vi "RSNRPZ Revision Query.vi"(8 "error in (no error)":errorcluster, 11 "VISA session":refnum<visa-resource-name> caption="VISA resource name") -> (0 "error out":errorcluster, 1 "Firmware Revision":string, 2 "Instrument Driver Revision":string, 3 "dup VISA session":refnum<visa-resource-name> caption="VISA resource name")   [LabVIEW 2010]
doc: "This VI returns the DRIVER revision (only). Although a parameter for the INSTRUMENT revision exists, the instrument revision is NOT set by this function, but an empty string is always returned for the instrument revision"
uses:
  rsnrpz_32.dll
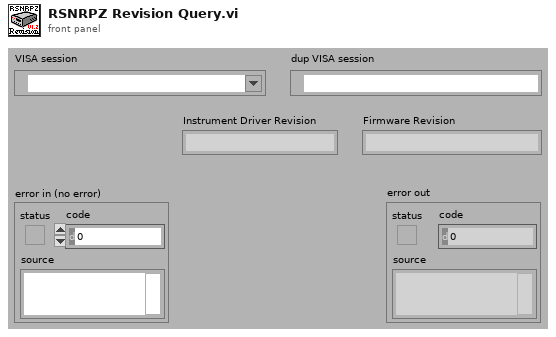
[diagram p1: front panel]
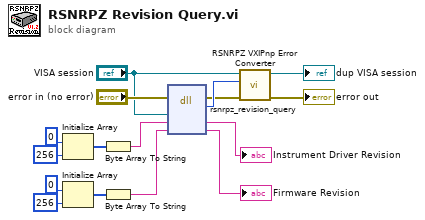
[diagram p0: block diagram]
diagram:
  n1 = Initialize Array(u8 0, 256) -> (w14:u8[])
  n2 = Initialize Array(u8 0, 256) -> (w11:u8[])
  n3 = Byte Array To String(unsigned byte array=w14) -> (string=w9:string)
  n4 = Byte Array To String(unsigned byte array=w11) -> (string=w7:string)
  n5 = dll-call lib="rsnrpz_32.dll" fn="rsnrpz_revision_query"(error in="error in (no error)", "VISA Session"="VISA session", "Instrument Driver Revision"=w9, "Firmware Revision"=w7) -> (error out=w5:errorcluster, "Status"=w10:i32, "Instrument Driver Revision"=→"Instrument Driver Revision":string, "Firmware Revision"=→"Firmware Revision":string)  [unwired: 3 in, 1 out]
  n6 = call <instrlib>:"RSNRPZ VXIPnp Error Converter.vi"("error in"=w5, "VXIPnp error code"=w10, "VISA session"="VISA session") -> ("error out"=→"error out":errorcluster, "dup VISA session"=→"dup VISA session":refnum<visa-resource-name>)  [unwired: 7 in]
